vi "Get Time Delta.vi"(2 "reference time (0)":dbl, 3 "anything in (for synchronization)":variant) -> (0 "time delta [s]":dbl, 1 "time now":dbl format="%_19f")   [LabVIEW 2020, in "GOLPI library.lvlib"]
doc: "Gets relative timestamp and eventually calculates delta time from reference timestamp. Use variant input to synchronize call with whatever signal."
uses:
  GOLPI library.lvlib
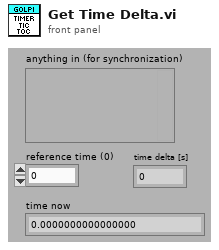
[diagram p1: front panel]
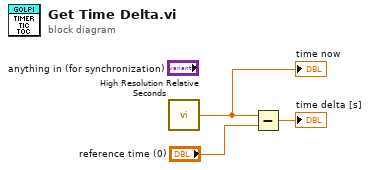
[diagram p0: block diagram]
diagram:
  n1 = call <vilib>:"High Resolution Relative Seconds.vi"() -> ("relative seconds"=w3:dbl)
  "time now" <- w3
  n2 = Subtract(x=w3, y="reference time (0)") -> (x-y=→"time delta [s]":dbl)
